vi "Write-Async-with-TypeResolving-Sensata.vi"() -> ()   [LabVIEW 2020]
doc: "ADS asynchronous write example using preconfigured blocks. \n\nThe client writes data asynchronously and does not wait for the respose from server."
uses:
  <userlib>/Beckhoff-LabVIEW-Interface/_DependsOn/TypeDefs/Low-Levels/Symbol Interface Mode.ctl
  <userlib>/Beckhoff-LabVIEW-Interface/_DependsOn/With TypeResolving/Write Async Single TypeResolved.vi
panel:
  in  "nVar":dbl format="%#_13g"
  out "Has Matched?":bool
  out "Iterations":i32
  in  "Symbol file path":path
  out "Write Status":bool
  # "The example starts with retrieving an\nADS Symbol. The symbol can be selected:\n- Using Symbol file in symbol file path\n- Using Symbol Interface (UI), which is opened automatically if file path is empty.\n\nThe example writes , only once, a double  value asynchronously to a LREAL variable located in TwinCAT3. Since the call is asynchronous, the example does not waits on ADS response. The example demonstrates how many iteration it takes to successfully write the value to TwinCAT3.\n\nThe example uses TypeResolver to check whether the selected ADS Symbol is of type LREAL or not.\n\nCheck Write status and bHasMached if write has succeeded.\n\nFor more information, please refer to block diagram comments."
  # "Note: This example is only an illustration of all possible ways how this Product can be used."
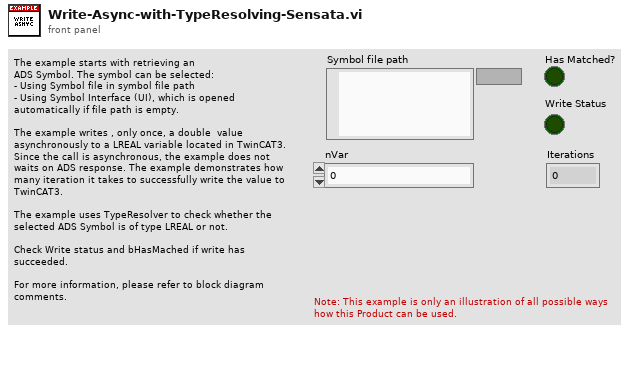
[diagram p1: front panel]
types:
  T1 = cluster{"nVar1":i16, "nVar2":u32, "sVar3":string[]}
  T2 = typedef "Symbol Interface Mode.ctl" = enum16{"Read Only", "Write Only", "Read & Write"}
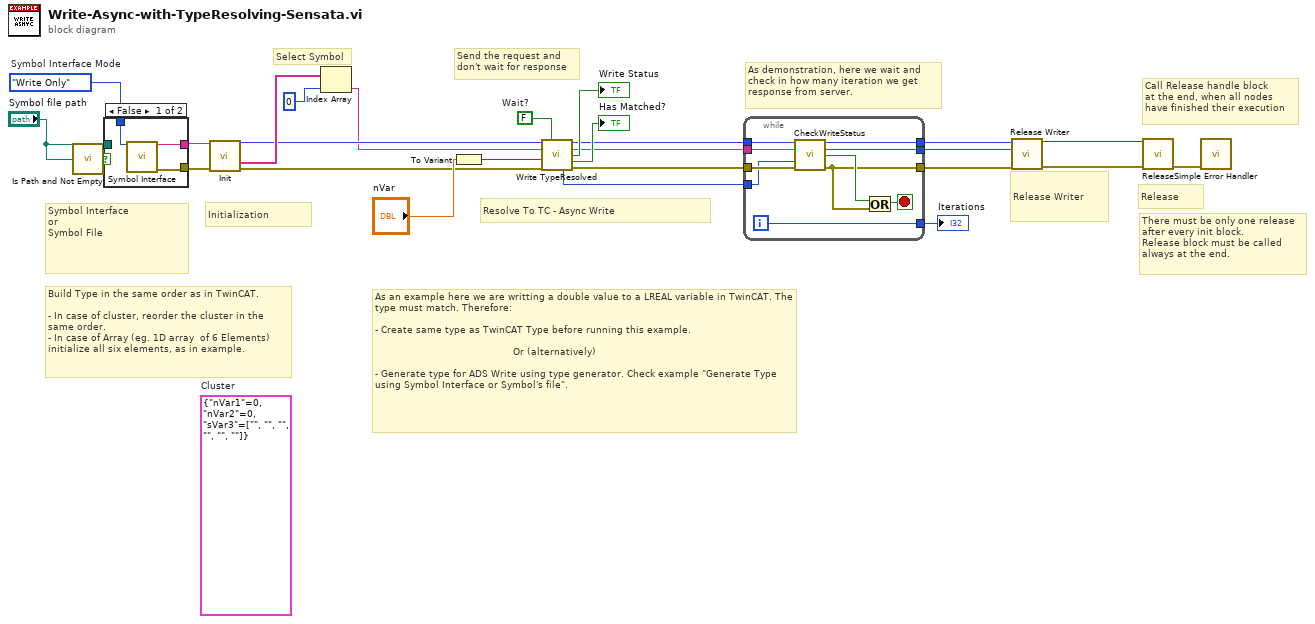
[diagram p0: block diagram]
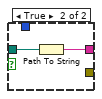
[diagram p2: hidden frame]
diagram:
  (unwired) T1 {"nVar1"=0, "nVar2"=0, "sVar3"=["", "", "", "", "", ""]}  # Cluster
  w2 = Symbol_Interface_Mode."Write Only"  # Symbol Interface Mode
  w18 = FALSE  # Wait?
  # "As an example here we are writting a double value to a LREAL variable in TwinCAT. The type must match. Therefore:\n\n- Create same type as TwinCAT Type before running this example. \n                                              \n                                              Or (alternatively)\n\n- Generate type for ADS Write using type generator. Check example \"Generate Type using Symbol Interface or Symbol's file\"."
  # "Build Type in the same order as in TwinCAT.\n\n- In case of cluster, reorder the cluster in the\nsame order.\n- In case of Array (eg. 1D array  of 6 Elements) \ninitialize all six elements, as in example."
  # "Symbol Interface\nor\nSymbol File"
  # "Send the request and\ndon't wait for response"
  # "Resolve To TC - Async Write"
  # "Release Writer"
  # "As demonstration, here we wait and \ncheck in how many iteration we get\nresponse from server."
  # "Call Release handle block\nat the end, when all nodes\nhave finished their execution"
  # "There must be only one release\nafter every init block.\nRelease block must be called\nalways at the end."
  # "Select Symbol"
  # "Release"
  # "Initialization"
  n1 = call <vilib>:"Is Path and Not Empty.vi"("path"="Symbol file path") -> ("Is Path and Not Empty?"=w6:bool)  [unwired: 4 in]
  n2 = case shown="False" w6 {
    tunnel: [w29 w31] -> w5
    tunnel: "Symbol file path" -> [_ w30]
    tunnel: [w28 _] -> w4
    tunnel: w2 -> [w27 _]
    frame False {
      n3 = call <userlib>:"Symbol Interface.vi"("Symbol Interface Mode"=w27) -> ("PortInfo"=w29:string, "error out"=w28:errorcluster)  [unwired: 13 in]
    }
    frame True {
      n4 = Path To String(path=w30) -> (string=w31:string)
    }
  }
  n5 = call <userlib>:"Init.vi"("XMLDescription"=w5, "error in (no error)"=w4) -> ("Handle"=w17:u32, "WriteGrpSymbols"=w25:string[], "error out"=w16:errorcluster)  [unwired: 9 in, 2 out]
  n6 = Index Array(array=w25, index=0) -> (element=w11:string)
  n7 = To Variant(anything="nVar") -> (Variant=w19:variant)
  n8 = call-poly <userlib>:"Write TypeResolved.vi"("Handle"=w17, "Wait?"=w18, "SymbolName"=w11, "WData"=w19, "error constant"=w16) -> ("Handle"=w13:u32, "SymbolName"=w9:string, "Write Status?"=→"Write Status":bool, "Has Matched?"=→"Has Matched?":bool, "WriteHandle"=w8:u32, "error out"=w12:errorcluster)  [unwired: 5 in]
  n9 = while {
    tunnel: [w39] -> w23
    tunnel: [w38] -> w24
    tunnel: [w37] -> w21
    tunnel: w13 -> [w36]
    tunnel: w12 -> [w35]
    tunnel: [w34] -> w10
    tunnel: w9 -> [w33]
    tunnel: w8 -> [w32]
    i -> [w37]
    stop <- w41 stop-if-true
    n10 = call <userlib>:"CheckWriteStatus.vi"("Handle"=w36, "SymbolName"=w33, "WriteHandle"=w32, "error in"=w35) -> ("Handle"=w34:u32, "WriteHandle"=w38:u32, "Write status?"=w40:bool, "error out"=w39:errorcluster)  [unwired: 8 in]
    n11 = Or(x=w40, y=w39) -> (x .or. y?=w41:bool)
  }
  "Iterations" <- w21
  n12 = call <userlib>:"Release Writer.vi"("Handle"=w10, "WriteHandle"=w24, "error in (no error)"=w23) -> ("Handle"=w22:u32, "error out"=w7:errorcluster)  [unwired: 11 in]
  n13 = call <userlib>:"Release.vi"("Handle"=w22, "error in (no error)"=w7) -> ("error out"=w1:errorcluster)  [unwired: 13 in]
  n14 = call <vilib>:"Simple Error Handler.vi"("error in (no error)"=w1) -> ()  [unwired: 4 in, 5 out]
